vi "Test Copy All Paths.vi"(8 "error in (no error)":errorcluster) -> (0 "error out":errorcluster)   [LabVIEW 2019]
uses:
  Setting Database/Setting Database.lvclass
  C:/Program Files (x86)/National Instruments/LabVIEW 2019/vi.lib/JKI/JKI SMO/SMO/SMO.lvclass
  Setting Database/Typedefs/PrivateEvents--Setting Database.CopyActivePathToAll.ctl
  ObjectSettings/ObjectSettings.lvclass/ObjectSettings.ctl
  ObjectSettings/Accessors/Read Enabled.vi
  ObjectSettings/Accessors/Write Enabled.vi
  Path Settings/Path Settings.lvclass
  C:/Users/Albro/Documents/GitHub/AFM-Lithography/lvsrc/Classes/Settings/ObjectSettings/ObjectSettings.lvclass
  <vilib>/addons/_JKI Toolkits/Caraya/classes/Assert/Assert Equal Value_Variant.vi
  <vilib>/addons/_JKI Toolkits/Caraya/classes/Assert/Assert Not Error.vi
  <vilib>/addons/_JKI Toolkits/Caraya/classes/Test/Test.lvclass
  <vilib>/addons/_JKI Toolkits/Caraya/classes/Assert/Assert.lvclass
  <vilib>/JKI/JKI SMO/SMO/SMO.lvclass
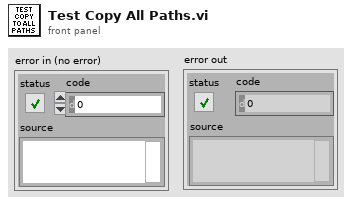
[diagram p1: front panel]
types:
  T1 = typedef "Setting Database.lvclass/PrivateEvents--Setting Database.CopyActivePathToAll.ctl" = bool
  T2 = typedef "Setting Database.lvclass/PublicEvents--Cluster.ctl" = cluster{"NewActivePath":refnum<user-event>, "PathsUpdated":refnum<user-event>, "RectanglesUpdated":refnum<user-event>, "NewActiveRectangle":refnum<user-event>, "NewActiveFunnel":refnum<user-event>, "FunnelsUpdated":refnum<user-event>, "NewActiveDot":refnum<user-event>, "DotsUpdated":refnum<user-event>}
  T3 = typedef "Setting Database.lvclass/PrivateEvents--Setting Database.Refresh.ctl" = cluster{"Paths":string[], "Rectangles":string[], "Funnels":string[], "Dots":string[]}
  T4 = typedef "Setting Database.lvclass/PublicEvents--Setting Database.NewActivePath.ctl" = refnum<class "Path Settings.lvclass">
  T5 = typedef "Setting Database.lvclass/PublicEvents--Setting Database.PathsUpdated.ctl" = refnum<class "Path Settings.lvclass">[]
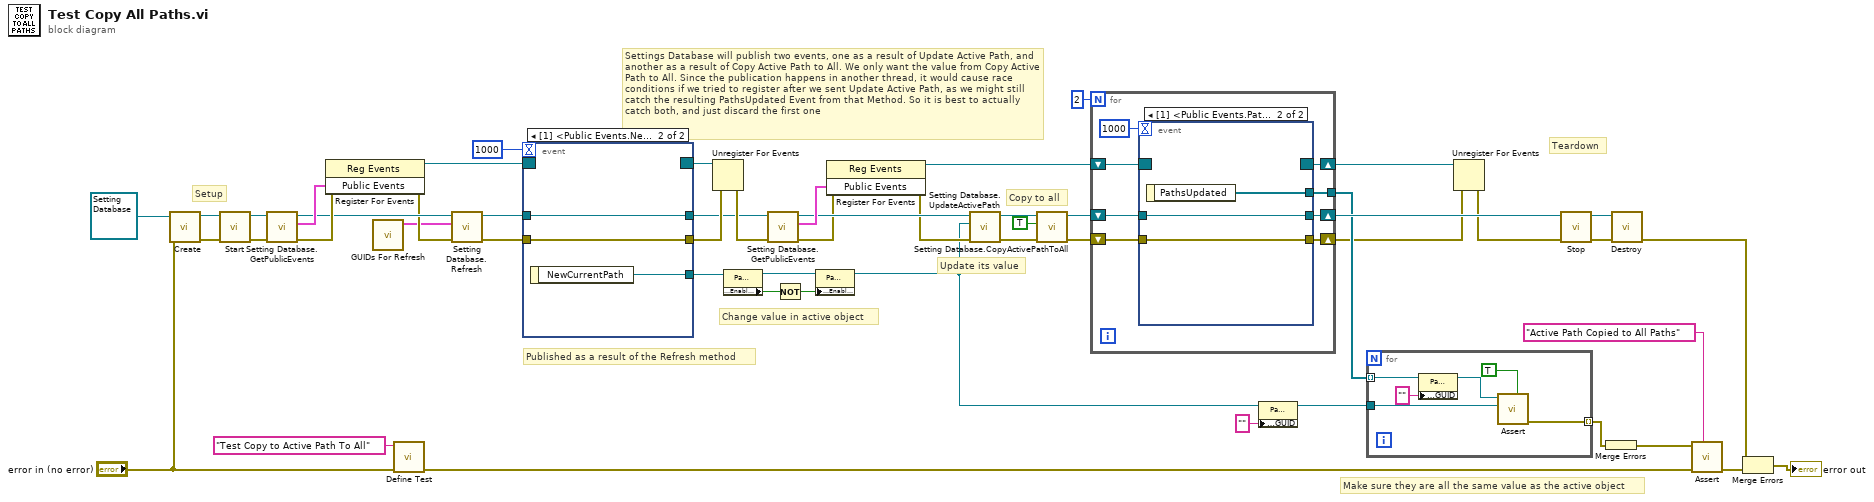
[diagram p0: block diagram]
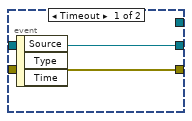
[diagram p2: hidden frame]
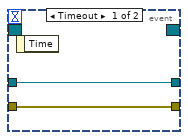
[diagram p3: hidden frame]
diagram:
  # "Make sure they are all the same value as the active object"
  # "Copy to all"
  # "Update its value"
  # "Change value in active object"
  # "Published as a result of the Refresh method"
  # "Settings Database will publish two events, one as a result of Update Active Path, and another as a result of Copy Active Path to All. We only want the value from Copy Active Path to All. Since the publication happens in another thread, it would cause race conditions if we tried to register after we sent Update Active Path, as we might still catch the resulting PathsUpdated Event from that Method. So it is best to actually catch both, and just discard the first one"
  # "Teardown"
  # "Setup"
  n1 = call <vilib>:"Create.vi"("error in (no error)"="error in (no error)", "SMO"=refnum<class "Setting Database.lvclass"> refnum ("Setting Database.lvclass")) -> ("error out"=w49:errorcluster, "SMO out"=w40:refnum<class "Setting Database.lvclass">)  [unwired: 7 in, 1 out]
  n2 = call <vilib>:"Start.vi"("error in (no error)"=w49, "SMO"=w40) -> ("error out"=w48:errorcluster, "SMO out"=w39:refnum<class "Setting Database.lvclass">)  [unwired: 8 in]
  n3 = call "Setting Database.GetPublicEvents.vi"("error in (no error)"=w48, "Setting Database"=w39) -> ("error out"=w45:errorcluster, "Public Events"=w34:T2, "Setting Database out"=w32:refnum<class "Setting Database.lvclass">)  [unwired: 7 in]
  n4 = register-events(error in=w45, w34) -> (reference out=w35:refnum<event-registration>, error out=w31:errorcluster)  [unwired: 1 in]
  n5 = call "GUIDs For Refresh.vi"() -> ("Initialize"=w4:T3)  [unwired: 11 in]
  n6 = call <vilib>:"Define Test.vi"("error in (no error)"="error in (no error)", "Label (VI Title)"="Test Copy to Active Path To All") -> ("error out"=w51:errorcluster)  [unwired: 8 in, 1 out]
  n7 = call "Setting Database.Refresh.vi"("error in (no error)"=w31, "Initialize"=w4, "Setting Database"=w32) -> ("error out"=w30:errorcluster, "Setting Database out"=w29:refnum<class "Setting Database.lvclass">)  [unwired: 7 in]
  n8 = event shown="[1] <Public Events.NewActivePath>: User Event" {
    selector: w35 -> [_ _]
    dyn-events: [_ _] -> w37
    timeout: 1000 -> [_ _]
    tunnel: [w54 w57] -> w46
    tunnel: w30 -> [w54 w57]
    tunnel: w29 -> [w53 w56]
    tunnel: [w53 w56] -> w14
    tunnel: [_ w55] -> w28
    event Timeout {
      n9 = event-data() -> ()  [unwired: 1 in, 1 out]
    }
    event User Event {
      n10 = event-data() -> ("NewCurrentPath"=w55:T4)  [unwired: 1 in]
    }
  }
  n11 = Unregister For Events(event registration refnum=w37, error in=w46) -> (error out=w15:errorcluster)
  n12 = property class="Path Settings.lvclass"(reference=w28) -> (reference out=w27:T4, "Accessors:Enabled"=w26:bool)  [unwired: 1 in, 1 out]
  n13 = call "Setting Database.GetPublicEvents.vi"("error in (no error)"=w15, "Setting Database"=w14) -> ("error out"=w10:errorcluster, "Public Events"=w23:T2, "Setting Database out"=w13:refnum<class "Setting Database.lvclass">)  [unwired: 7 in]
  n14 = Not(x=w26) -> (.not. x?=w25:bool)
  n15 = property class="Path Settings.lvclass"(reference=w27, "Accessors:Enabled"=w25) -> (reference out=w2:T4)  [unwired: 1 in, 1 out]
  n16 = register-events(error in=w10, w23) -> (reference out=w19:refnum<event-registration>, error out=w9:errorcluster)  [unwired: 1 in]
  n17 = call "Setting Database.UpdateActivePath.vi"("error in (no error)"=w9, "UpdateCurrentPath"=w2, "Setting Database"=w13) -> ("error out"=w11:errorcluster, "Setting Database"=w12:refnum<class "Setting Database.lvclass">)  [unwired: 7 in]
  n18 = call "Setting Database.CopyActivePathToAll.vi"("error in (no error)"=w11, "CopyActiveToAll"=T1 TRUE, "Setting Database"=w12) -> ("error out"=w20:errorcluster, "Setting Database out"=w22:refnum<class "Setting Database.lvclass">)  [unwired: 7 in]
  n19 = for {
    N: 2 -> [_]
    tunnel: [w60] -> w18
    shift-right: [w64] -> w21
    shift-left: w22 -> [w65]
    shift-right: [w63] -> w6
    shift-left: w20 -> [w62]
    shift-right: [w59] -> w7
    shift-left: w19 -> [w61]
    n20 = event shown="[1] <Public Events.PathsUpdated>: User Event" {
      selector: w61 -> [_ _]
      dyn-events: [_ _] -> w59
      timeout: 1000 -> [_ _]
      tunnel: w65 -> [w67 w70]
      tunnel: [w67 w70] -> w64
      tunnel: [w66 w69] -> w63
      tunnel: w62 -> [w66 w69]
      tunnel: [_ w68] -> w60
      event Timeout {
        n21 = event-data() -> ()  [unwired: 1 in, 3 out]
      }
      event User Event {
        n22 = event-data() -> ("PathsUpdated"=w68:T5)  [unwired: 1 in]
      }
    }
  }
  n23 = property class="Path Settings.lvclass"(reference=w2, "Accessors:GUID"="" ("GUID")) -> (reference out=w1:T4)  [unwired: 1 in, 1 out]
  n24 = for {
    tunnel: w18 -> [w71] mode=indexing
    tunnel: w1 -> [w76]
    tunnel: [w75] -> w17 mode=indexing
    n25 = property class="Path Settings.lvclass"(reference=w71, "Accessors:GUID"="" ("GUID")) -> (reference out=w72:refnum<class "Path Settings.lvclass">)  [unwired: 1 in, 1 out]
    n26 = call-poly <vilib>:"Assert.vi"("Assert Only? (F)"=TRUE, "Actual"=w76, "Expected"=w72) -> ("error out"=w75:errorcluster)  [unwired: 7 in, 1 out]
  }
  n27 = Unregister For Events(event registration refnum=w7, error in=w6) -> (error out=w5:errorcluster)
  n28 = call <vilib>:"Stop.vi"("error in (no error)"=w5, "SMO"=w21) -> ("error out"=w47:errorcluster, "SMO out"=w38:refnum<class "Setting Database.lvclass">)  [unwired: 8 in]
  n29 = Merge Errors(w17) -> (w16:errorcluster)
  n30 = call <vilib>:"Destroy.vi"("error in (no error)"=w47, "SMO"=w38) -> ("error out"=w44:errorcluster)  [unwired: 9 in]
  n31 = call-poly <vilib>:"Assert.vi"("Label"="Active Path Copied to All Paths" ("Label (VI Title)"), "error in (no error)"=w51, "Not Error?"=w16) -> ("error out"=w52:errorcluster)  [unwired: 7 in, 1 out]
  n32 = Merge Errors(w44, w52) -> (→"error out":errorcluster)
